vi "validate configuration.vi"(8 "error in":errorcluster, 11 "Shared Library Module configuration in":refnum<class "Shared Library Module configuration.lvclass">) -> (0 "error out":errorcluster, 3 "Shared Library Module configuration out":refnum<class "Shared Library Module configuration.lvclass">)   [LabVIEW 2013, in "Shared Library Module configuration.lvclass"]
doc: "This function performs validation of the configuration. This function should be safe to call at any point and should not rely on anything in the runtime environment.Platypus Framework 1.0.1.60\nNI Systems Engineering - National Instruments"
uses:
  Shared Library Module configuration.lvclass
  <vilib>/NI/Tag Bus Module Framework/module configuration/TBM module configuration.lvclass
  Shared Library Module configuration.lvclass/Shared Library Module configuration.ctl
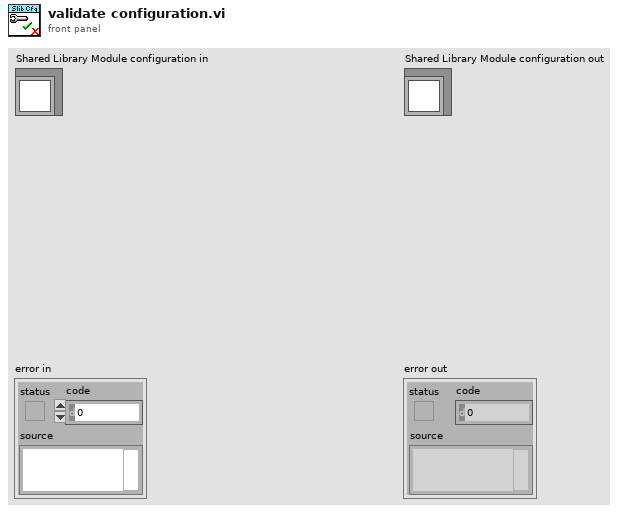
[diagram p1: front panel]
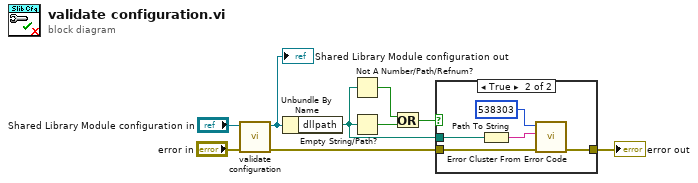
[diagram p0: block diagram]
diagram:
  n1 = call-parent "validate configuration.vi"("error in"="error in", "configuration in"="Shared Library Module configuration in") -> ("error out"=w2:errorcluster, "configuration out"=w3:refnum<class "Shared Library Module configuration.lvclass">)  [unwired: 8 in]
  "Shared Library Module configuration out" <- w3
  n2 = Unbundle By Name(w3) -> ("dllpath"=w4:path)
  n3 = Not A Number/Path/Refnum?(number/path/refnum=w4) -> (NaN/Path/Refnum?=w6:bool)
  n4 = Empty String/Path?(string/path=w4) -> (empty?=w7:bool)
  n5 = Or(x=w6, y=w7) -> (x .or. y?=w5:bool)
  n6 = case shown="True" w5 {
    tunnel: [w10 w14] -> w1
    tunnel: w2 -> [w10 w15]
    tunnel: w4 -> [_ w12]
    frame False {
    }
    frame True {
      n7 = Path To String(path=w12) -> (string=w11:string)
      n8 = call <vilib>:"Error Cluster From Error Code.vi"("error in (no error)"=w15, "error message (\"\")"=w11, "error code (0)"=538303) -> ("error out"=w14:errorcluster)  [unwired: 6 in]
    }
  }
  "error out" <- w1
